vi "Evegeny.vi"() -> ()   [LabVIEW 2017]
panel:
  out "result string":string
  out "string 2":string
  out "array w/ subset deleted":u8[](array[numeric]) format="%.0x"
  out "unsigned byte array":u8[](array[numeric]) format="%.0x"
  out "x = y? 2":bool[](array[boolean])
  out "deleted portion":u8[](array[numeric]) format="%.0x"
  in  "string":string
  out "subarray":u8[](array[numeric]) format="%.0x"
  in  "y":u16=21045 format="%.0x"
  out "x = y?":bool
  out "Bytes":i32
  out "CheckSum":u16 format="%.0x"
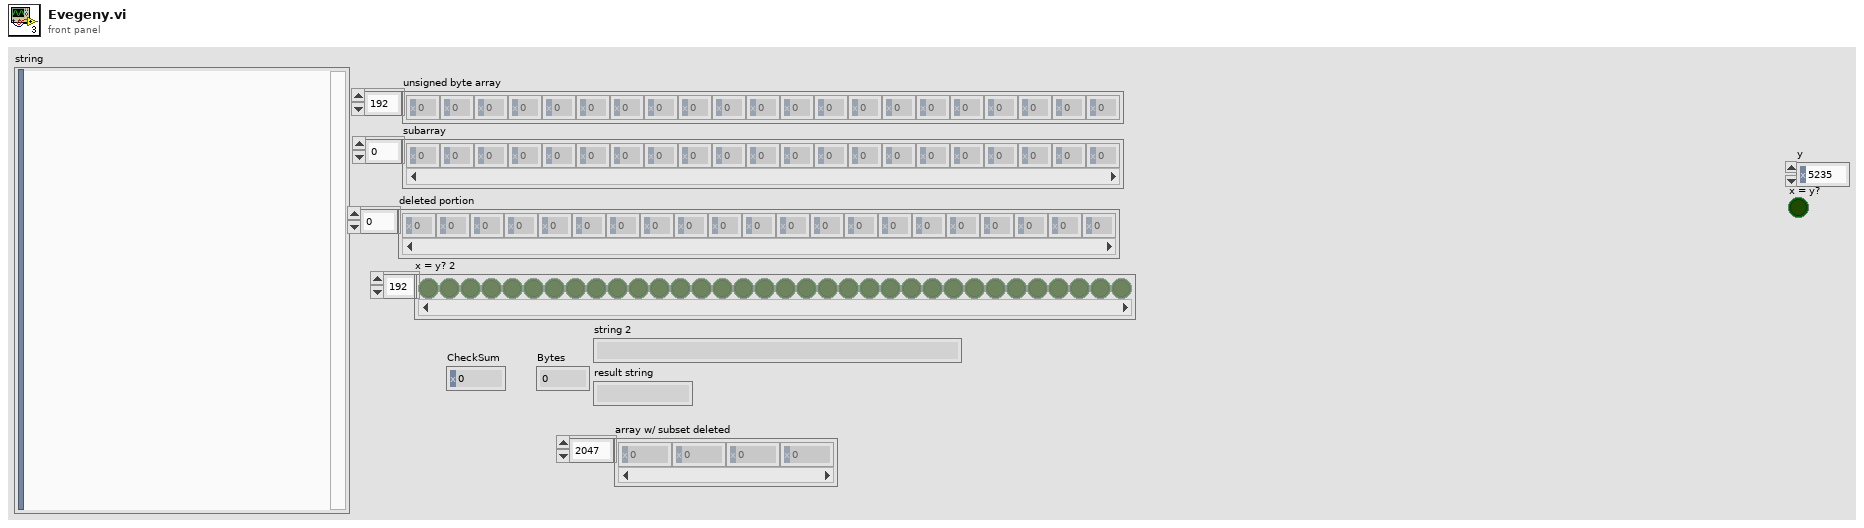
[diagram p1: front panel]
diagram:
  w17 = u8[][] array8x55236[441888 elements] ("Array 5")
  n1 = Index Array(array=w17, index (row)=3) -> (element=w15:u8[])  [unwired: 1 in]
  "subarray" <- w15
  n2 = Index Array(array=w17, index (row)=3) -> (element=w20:u8[])  [unwired: 1 in]
  n3 = String To Byte Array(string="string") -> (unsigned byte array=w11:u8[])
  "unsigned byte array" <- w11
  n4 = Delete From Array(array=w15, length=12294, index=0) -> (array with subset deleted=w9:u8[])  [unwired: 1 out]
  "deleted portion" <- w9
  n5 = Delete From Array(array=w20, length=2048, index=10246) -> ()  [unwired: 2 out]
  n6 = flat-sequence {
    tunnel: w11 -> [w24]
    frame #0 {
      n7 = for {
        tunnel: w24 -> [w39] mode=indexing
        shift-right: [w34] -> _
        shift-left: u8[] [] -> [w33]
        shift-right: [w27] -> w23
        shift-left: u16 0 -> [w32]
        tunnel: [w28] -> w22
        i -> [w38]
        stop <- w28 stop-if-true
        n8 = Split Number(x=w39) -> (hi(x)=w31:u8, lo(x)=w30:u8)
        n9 = Build Array(w31, w30) -> (w36:u8[])
        n10 = Compound Arithmetic op=ADD(w32, w31, w30) -> (w27:u16)
        n11 = Multiply(x=w38, y=2) -> (x*y=w35:i32)
        n12 = Equal?(x=w27, y="y") -> (x = y?=w28:bool)
        n13 = Insert Into Array(array=w33, index=w35, new element=w36) -> (w34:u8[])
        "Bytes" <- w38
      }
      "CheckSum" <- w23
      "x = y?" <- w22
    }
  }
  n14 = Equal?(x=w9, y=w11) -> (x = y?=→"x = y? 2":bool[])
  n15 = Delete From Array(array=w9, length=2048, index=0) -> (deleted portion=w6:u8[])  [unwired: 1 out]
  "array w/ subset deleted" <- w6
  n16 = Byte Array To String(unsigned byte array=w6) -> (string=→"string 2":string)
  n17 = Search and Replace String(replace all?=TRUE ("replace all? (F)"), input string="A4 88 7E 76 35 EA AD 5D AD 5C 8A DD 8E DC A5 88 A4 5C 7E 8F EA F8 7E 76 13 E1 AD 5C 8A DC A4 5C 7E 76 BE E9 1F 76 4A 02 A6 1E 16 02 14 07 A9 8A C4 C2 45 6F 18 02 E4 C4 1F 76 4A 02 14 07 A9 8A C4 C2 3D 6F 1A 02 E4 C4 1F 76 4A 02 14 07 A9 8A C4 C2 35 6F 03 9A 34 6F 45 92 01 52 97 61 02 52 C0 61 03 52 E8 61 04 52 EE 61 F5 6F 1F 76 4B 02 14 06 1F 76 74 02 04 1E 20 6F 1F 76 4B 02 16 06 1F 76 74 02 04 1E 19 6F 1F 76 4B 02 18 06 7E 76 A9 F9 1F 76 74 02 04 1E 10 6F 1F 76 4B 02 1A 06 1F 76 74 02 04 1E 09 6F 01 52 E1 61 02 52 E6 61 03 52 EB 61 04 52 F2 61 03 9A 02 6F 00 9A 8E FE 06 00 BD B2 0E FE 44 A8 D4 92 45 96 DC 40 ED FF 0F 01 EF FF CF 00 1F 76 7D 02 06 06 04 61 39 9A EF FF 15 01 E4 06 04 61 06 02 E4 0F 04 67 15 9A EF FF 0D 01 1C 02 1F 76 4A 02 14 07 A7 1E E4 92 C7 96 EF FF 03 01 E4 06 1F 76 60 02 12 1E 7E 76 A1 EA A6 1E 00 9A A8 28 70 42 42 1E A6 06 7E 76 88 E5 A6 1E 00 9A A8 28 7A 44 42 1E A6 06 7E 76 96 E1 44 8A A9 8B E4 06 7E 76 A1 EA 42 1E A9 B2 7E 76 96 E1 AD 5C 8E DC A4 88 7E 76 35 EA AD 5D AD 5C 8A DD 8E DC A5 88 A4 5C 7E 8F EA F8 7E 76 13 E1 AD 5C 8A DC A4 5C 7E 76 BE E9 1F 76 4A 02 A6 1E 1E 02 14 07 A9 8A C4 C2 EF FF C7 00 E4 06 1F 76 60 02 0C 1E 7E 76 A1 EA A6 1E 00 9A A8 28 70 42 42 1E A6 06 7E 76 88 E5 A6 1E 00 9A A8 28 7A 44 42 1E A6 06 7E 76 96 E1 1F 76 78 02 A9 8B 04 06 7E 76 A1 EA 42 1E A9 B2 7E 76 96 E1 AD 5C 8E DC A4 88 7E 76 35 EA AD 5D AD 5C 8A DD 8E DC A5 88 A4 5C 7E 8F EA F8 7E 76 13 E1 AD 5C 8A DC A4 5C 7E 76 BE E9 1F 76 4A 02 A6 1E 20 02 14 07 A9 8A C4 C2 EF FF 8A 00 E4 06 AD 5C 8E DC A4 88 7E 76 35 EA AD 5D AD 5C 8A DD 8E DC A5 88 A4 5C 7E 8F EA F8 7E 76 13 E1 AD 5C 8A DC A4 5C 7E 76 BE E9 1F 76 4A 02 A6 1E 22 02 14 07 A9 8A C4 C2 6C 6F E4 06 AD 5C 8E DC A4 88 7E 76 35 EA AD 5D AD 5C 8A DD 8E DC A5 88 A4 5C 7E 8F EA F8 7E 76 13 E1 AD 5C 8A DC A4 5C 7E 76 BE E9 1F 76 4A 02 A6 1E 24 02 14 07 A9 8A C4 C2 4F 6F 03 9A 4E 6F 03 52 0A 62 03 52 84 61 01 52 E1 FF 2E FF 02 52 E1 FF 43 FF F4 6F 04 52 B8 61 05 52 D3 61 EF 6F 1C 02 1F 76 4A 02 14 07 A9 8A 1F 76 74 02 C4 0E 04 1E 33 6F 1F 76 60 02 12 06 1F 76 74 02 04 1E 2C 6F 1F 76 60 02 0C 06 1F 76 74 02 04 1E 25 6F 22 02 1F 76 4A 02 14 07 A9 8A 1F 76 74 02 C4 06 04 1E 1B 6F 24 02 1F 76 4A 02 14 07 A9 8A 1F 76 74 02 C4 06 04 1E 11 6F 03 9A 10 6F 03 52 08 62 03 52 E0 61 01 52 CD 61 02 52 D5 61 F6 6F 04 52 E0 61 05 52 E8 61 F1 6F 00 9A 8E FE BE 8B 06 00 04 FE 42 A8 D4 92 43 96 DC 40 ED FF E8 00 79 6F A2 02 1F 76 4A 02 14 07 A9 8A C4 92 04 60 19 9A EF FF F2 00 42 8A 02 02 E4 0F 09 60 00 02 1F 76 77 02 28 1E BF 56 22 02 EF FF E5 00 01 02 E4 0F 07 60 1F 76 77 02 BF 56 22 06 EF FF DC 00 E4 06 07 60 1F 76 77 02 BF 56 22 05 EF FF D4 00 15 9A EF FF D2 00 A2 02 1F 76 4A 02 14 07 A7 1E E4 92 C7 96 EF FF C8 00 AE 02 E4 C4 1F 76 4A 02 14 07 A9 8A C4 C2 7E 76 A5 C5 EF FF BD 00 AC 02 E4 C4 1F 76 4A 02 14 07 A9 8A C4 C2 7E 76 A5 C5 EF FF B2 00 A8 02 E4 C4 1F 76 4A 02 14 07 A9 8A C4 C2 7E 76 A5 C5 EF FF A7 00 AA 02 E4 C4 1F 76 4A 02 14 07 A9 8A C4 C2 7E 76 A5 C5 EF FF 9C 00 A6 02 E4 C4 1F 76 4A 02 14 07 A9 8A C4 C2 7E 76 A5 C5 EF FF 91 00 A4 02 E4 C4 1F 76 4A 02 14 07 A9 8A C4 C2 7E 76 A5 C5 EF FF 86 00 03 9A EF FF 84 00 04 52 0C 62 04 52 CE 61 00 52 83 61 01 52 AB 61 02 52 B2 61 03 52 BB 61 F1 6F 05 52 CE 61 06 52 D7 61 07 52 E0 61 EA 6F 1F 76 77 02 22 92 08 52 08 60 1F 76 7D 02 06 06 1F 76 74 02 04 1E 62 6F 02 02 1F 76 74 02 04 1E 5D 6F A2 02 1F 76 4A 02 14 07 A9 8A 1F 76 74 02 C4 0E 04 1E 53 6F AE 02 1F 76 4A 02 14 07 A9 8A 1F 76 74 02 C4 06 04 1E 49 6F AC 02 1F 76 4A 02 14 07 A9 8A 1F 76 74 02 C4 06 04 1E 3F 6F A8 02 1F 76 4A 02 14 07 A9 8A 1F 76 74 02 C4 06 04 1E 35 6F AA 02 1F 76 4A 02 14 07 A9 8A 1F 76 74 02 C4 06 04 1E 2B 6F A6 02 1F 76 4A 02 14 07 A9 8A 1F 76 74 02 C4 06 04 1E 21 6F A4 02 1F 76 4A 02 14 07 A9 8A 1F 76 74 02 C4 06 04 1E 17 6F 03 9A 16 6F 04 52 0C 62 04 52 D3 61 00 52 A2 61 01 52 B1 61 02 52 B9 61 03 52 C1 61 F2 6F 05 52 D2 61 06 52 DA 61 07 52 E2 61 EB 6F 00 9A 84 FE 06 00 06 FE 42 1E 46 1E 1F 76 78 02 00 06 02 03 44 1E 01 3B 42 06 4A 03 A6 1E 44 06 40 FF A7 1E A6 06 A7 0F 05 65 42 06 44 03 46 1E 0E 6F 42 06 4A 03 A6 1E 44 06 40 FF 54 FF A7 1E A6 06 A7 0F 04 63 44 06 42 07 46 1E 46 06 86 FE 06 00 06 FE 46 1E 44 A8 4A 06 C4 1E 46 C4 08 02 44 07 A9 8A C4 C2 08 02 44 07 A9 8A 44 83 C4 06 44 8A C5 03 D4 1E 44 8A D4 C4 AC 28 1F 00 01 3B A6 06 22 56 A6 07 40 FF C4 07 F4 1E 00 BE 0C 02 44 07 A9 8A C4 C2 10 02 44 07 A9 8A C4 C2 44 8A 00 02 E4 1E 86 FE 06 00 08 FE 00 02 1F 76 79 02 08 1E 0A 1E 06 1E 14 1E 12 1E 0E 1E 1F 76 60 02 12 06 1F 76 79 02 10 1E 1F 76 60 02 0C 06 1F 76 79 02 16 1E 1F 76 6E 02 2A 06 1F 76 78 02 42 1E 00 06 44 1E 02 06 1F 76 60 02 46 1E 16 06 7E 76 6E B5 48 1E 1F 76 6E 02 00 8F 98 9E 2A 06 42 1E 48 06 7E 76 BA 9A 1F 76 7A 02 18 06 2A 1E 1F 76 79 02 18 1E 1F 76 7A 02 02 02 1A 0F 06 63 1F 76 79 02 BF 56 01 01 0B 6F 1A 0F 06 65 1F 76 79 02 BF 56 01 04 04 6F 1F 76 79 02 01 2B 88 FE 06 00 1F 76 79 02 06 06 06 65 BF 56 01 0A BF 56 02 09 05 6F BF 56 01 0B BF 56 02 09 06 00 04 FE 44 A8 42 1E 1F 76 79 02 06 06 06 65 BF 56 01 0A BF 56 02 08 05 6F BF 56 01 0B BF 56 02 08 1F 76 4B 02 BF 56 1C 02 84 FE 06 00 12 FE 51 7D 46 A8 44 1E 12 02 46 07 A9 8A C4 06 42 1E 44 06 7E 76 94 9A 50 1E 51 92 E1 FF 28 01 12 02 46 07 A9 8A 50 06 C4 03 48 1E 0A 02 46 07 A9 8A 46 83 C4 06 C5 03 4E 1E 12 02 46 07 A9 8A C4 06 C5 03 4A 1E 0E 02 46 07 A6 1E 12 02 46 07 A9 8A C4 06 A6 8A C4 03 4C 1E EF FF 09 01 48 06 08 63 1F 76 79 02 BF 56 01 0A BF 56 02 08 1C 6F 4A 06 48 0F 08 65 1F 76 79 02 BF 56 01 0A BF 56 02 08 12 6F 46 8A C4 06 42 1E 46 8A 50 06 7E 76 BA 9A 0A 02 46 07 A9 8A 48 06 C4 07 A6 1E 0A 02 46 07 A9 8A C4 C2 50 C4 08 02 46 07 A9 8A C4 C2 EF FF F5 00 48 06 09 63 1F 76 79 02 BF 56 01 0A BF 56 02 08 EF FF EB 00 4E 06 48 0F 09 65 1F 76 79 02 BF 56 01 0A BF 56 02 08 EF FF E0 00 46 8A C4 06 42 1E 46 8A 50 06 7E 76 BA 9A 0A 02 46 07 A9 8A 48 06 C4 07 A6 1E 0A 02 46 07 A9 8A C4 C2 EF FF CD 00 48 06 09 63 1F 76 79 02 BF 56 01 0A BF 56 02 08 EF FF C3 00 4E 06 4C 03 48 0F 09 65 1F 76 79 02 BF 56 01 0A BF 56 02 08 EF FF B7 00 12 02 46 07 A9 8A C4 06 46 8A 4E 03 4C 07 C4 1E 46 8A C4 06 42 1E 46 8A 50 06 7E 76 BA 9A 00 40 00 00 03 00 00 00 01 00 00 00 02 00 00 00 1F 76 79 02 BF 56 01 0B ", search string=" ") -> (result string=→"result string":string)  [unwired: 5 in, 3 out]
